vi "VisualizationCleanUp.vi"(8 "error in (no error)":errorcluster, 10 "ModuleRunningNormally?":bool, 11 "Module Name in":string) -> (0 "error out":errorcluster)   [LabVIEW 2018]
uses:
  VisualizationManagerActions.ctl
  NistPluggableModules/Visualization/VisualizeBase/VisualizeBase_class/VisualizeBase.lvclass
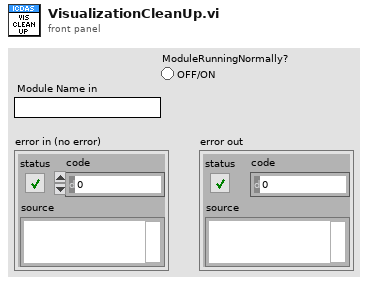
[diagram p1: front panel]
types:
  T1 = typedef "VisualizationManagerActions.ctl" = enum16{"Set", "LoadModVI", "PopInOutModVI", "Add", "Clear", "CloseVisMod", "LoadLatestModule", "Get"}
  T2 = typedef "OpenVisualizationVIs.ctl" = cluster{"Module Name":string, "VI ref":refnum<vi>, "In SubPanel?":bool, "Time Stamp":timestamp}
  T3 = enum32{"Bad", "Idle", "Run top level", "Running"}
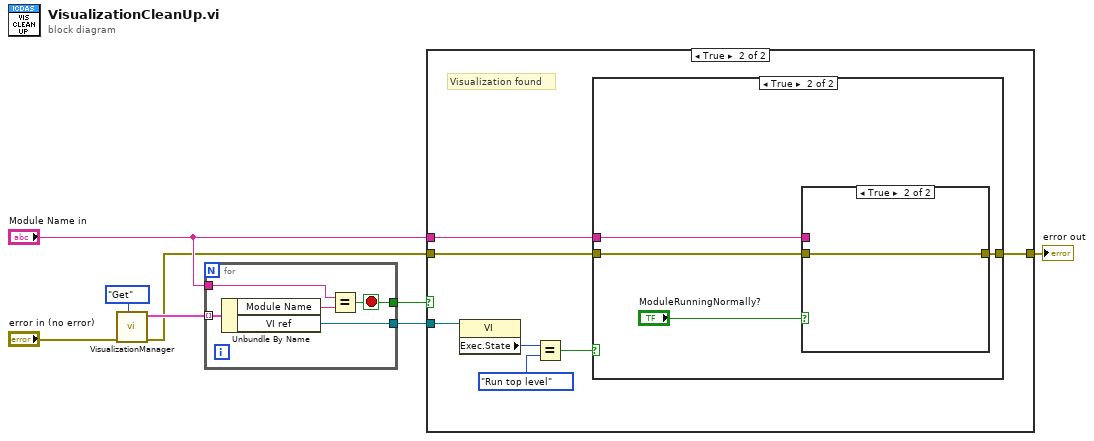
[diagram p0: block diagram]
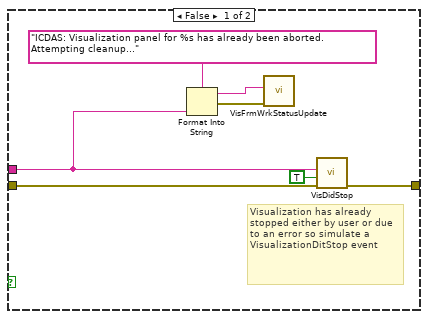
[diagram p3: hidden frame]
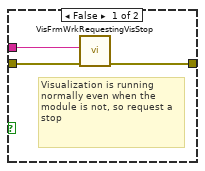
[diagram p4: hidden frame]
diagram:
  n1 = call "VisualizationManager.vi"("Action"=VisualizationManagerActions."Get", "error in (no error)"="error in (no error)") -> ("error out"=w1:errorcluster, "Open Visualization VIs out"=w6:T2[])  [unwired: 6 in, 2 out]
  n2 = for {
    tunnel: "Module Name in" -> [w12]
    tunnel: w6 -> [w13] mode=indexing
    tunnel: [w10] -> w7
    tunnel: [w9] -> w8
    stop <- w9 stop-if-true
    n3 = Unbundle By Name(w13) -> ("Module Name"=w11:string, "VI ref"=w10:refnum<vi>)
    n4 = Equal?(x=w12, y=w11) -> (x = y?=w9:bool)
  }
  n5 = case shown="True" w8 {
    tunnel: w1 -> [w14 w21]
    tunnel: [w14 w20] -> w3
    tunnel: "Module Name in" -> [_ w19]
    tunnel: w7 -> [_ w18]
    frame False {
      # "Visualization not found so don't do anything"
    }
    frame True {
      # "Visualization found"
      n6 = property class="VI"(reference=w18) -> ("Exec.State"=w17:T3)  [unwired: 1 in, 2 out]
      n7 = Equal?(x=w17, y=T3."Run top level") -> (x = y?=w15:bool)
      n8 = case shown="True" w15 {
        tunnel: w21 -> [w27 w32]
        tunnel: [w26 w31] -> w20
        tunnel: w19 -> [w22 w30]
        frame False {
          # "Visualization has already stopped either by user or due to an error so simulate a VisualizationDitStop event"
          n9 = Format Into String(format string="ICDAS: Visualization panel for %s has already been aborted. Attempting cleanup...", w22) -> (resulting string=w25:string, error out=w24:errorcluster)  [unwired: 2 in]
          n10 = call "VisFrmWrkStatusUpdate.vi"("error in (no error)"=w24, "Status"=w25) -> ()  [unwired: 9 in, 1 out]
          n11 = call "VisDidStop.vi"("error in (no error)"=w27, "DidStop?"=TRUE, "Module Name"=w22) -> ("error out"=w26:errorcluster)  [unwired: 8 in]
        }
        frame True {
          n12 = case shown="True" "ModuleRunningNormally?" {
            tunnel: w32 -> [w35 w36]
            tunnel: [w34 w36] -> w31
            tunnel: w30 -> [w33 _]
            frame False {
              # "Visualization is running normally even when the module is not, so request a stop"
              n13 = call "VisFrmWrkRequestingVisStop.vi"("error in (no error)"=w35, "VisualizationPluginNameToStop"=w33) -> ("error out"=w34:errorcluster)  [unwired: 9 in]
            }
            frame True {
            }
          }
        }
      }
    }
  }
  "error out" <- w3
